vi "LSX Set Factor Mode.vi"(5 "dA":dbl, 6 "dZ":dbl, 7 "dY":dbl, 8 "error in (no error)":errorcluster, 9 "dX":dbl, 10 "bAFactorMode":i32, 11 "lLSID":i32) -> (0 "error out":errorcluster, 3 "function return":i32)   [LabVIEW 2018, in "Tango.lvlib"]
doc: "TANGOAPI int TANGOCALL LSX_SetFactorMode (int lLSID, BOOL bAFactorMode, double dX, double dY, double dZ, double dA);"
uses:
  Tango.lvlib
  SubVIs/Tango_DLL.dll
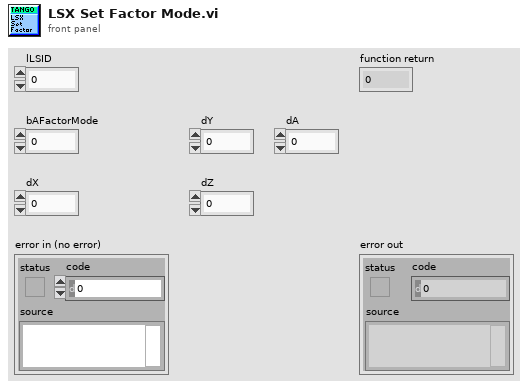
[diagram p1: front panel]
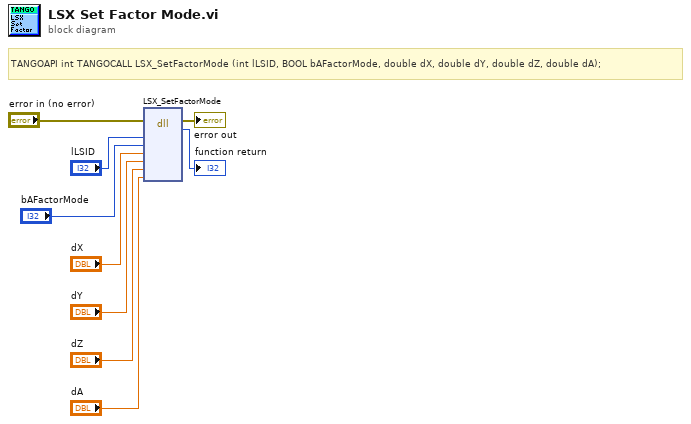
[diagram p0: block diagram]
diagram:
  # "TANGOAPI int TANGOCALL LSX_SetFactorMode (int lLSID, BOOL bAFactorMode, double dX, double dY, double dZ, double dA);"
  n1 = dll-call lib="C:/Users/Familie/Documents/LabviewIX81/lib/TANGO Stage/SubVIs/Tango_DLL.*" fn="LSX_SetFactorMode"(error in="error in (no error)", "lLSID"="lLSID", "bAFactorMode"="bAFactorMode", "dX"="dX", "dY"="dY", "dZ"="dZ", "dA"="dA") -> (error out=→"error out":errorcluster, →"function return":i32)  [unwired: 8 in, 1 out]
